vi "StopVI.vi"(0 "Application Ref in":refnum<vi>, 5 "VI in":refnum<vi>, 11 "error in (no error)":errorcluster) -> (15 "error out":errorcluster)   [LabVIEW 2016, in "Car Wash Test.lvlib"]
uses:
  Car Wash Test.lvlib
  APIs/Stimulus/VI/OpenVIFrontPanel.vi
  apis/Stimulus/KeyBoardSimulation/ValueSignalLatchBooleanString.vi
  Drona.lvlib
  apis/Stimulus/KeyBoardSimulation/KeyboardSimulation.lvlib
  apis/Stimulus/VI/VI.lvlib
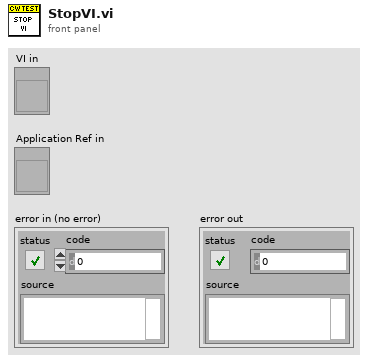
[diagram p1: front panel]
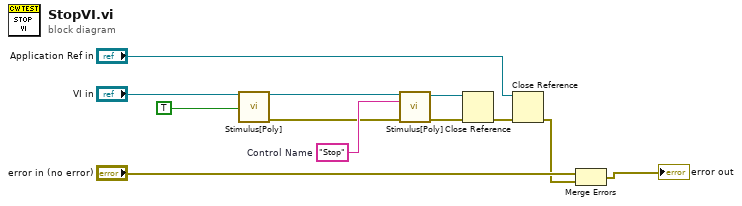
[diagram p0: block diagram]
diagram:
  w9 = "Stop"  # Control Name
  n1 = call-poly "Stimulus[Poly].vi"("VI Reference In"="VI in", "Wait Until Done (F)"=TRUE) -> ("VI Reference Out"=w3:refnum<vi>, "error out"=w1:errorcluster)  [unwired: 12 in]
  n2 = call-poly "Stimulus[Poly].vi"("VI Reference In"=w3, "Control Path"=w9, "error in"=w1) -> ("VI Reference Out"=w6:refnum<vi>, "error out"=w8:errorcluster)  [unwired: 11 in]
  n3 = Close Reference(reference=w6, error in (no error)=w8) -> (error out=w7:errorcluster)
  n4 = Close Reference(reference="Application Ref in", error in (no error)=w7) -> (error out=w5:errorcluster)
  n5 = Merge Errors("error in (no error)", w5) -> (→"error out":errorcluster)
